vi "Start Laser.vi"(8 "error in (no error)":errorcluster, 11 "Sim Laser Driver in":refnum<class "Sim Laser Driver.lvclass">) -> (0 "error out":errorcluster, 3 "Sim Laser Driver out":refnum<class "Sim Laser Driver.lvclass">)   [LabVIEW 2022 SP3, in "Sim Laser Driver.lvclass"]
uses:
  Sim Laser Driver.lvclass
  Sim Laser Driver.lvclass/Sim Laser Driver.ctl
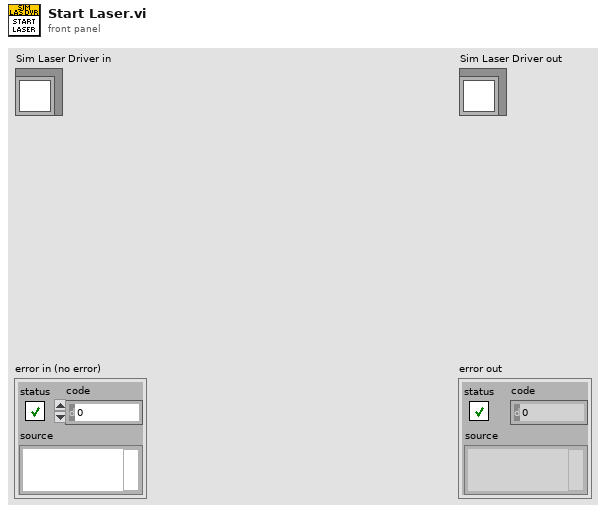
[diagram p1: front panel]
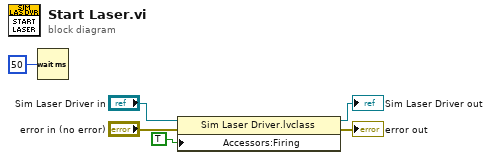
[diagram p0: block diagram]
diagram:
  n1 = Wait (ms)(milliseconds to wait=u32 50) -> ()  [unwired: 1 out]
  n2 = property class="Sim Laser Driver.lvclass"(reference="Sim Laser Driver in", error in="error in (no error)", "Accessors:Firing"=TRUE ("Firing")) -> (reference out=→"Sim Laser Driver out":refnum<class "Sim Laser Driver.lvclass">, error out=→"error out":errorcluster)
